vi "Append Image to Report (path).vi"(0 "report in":refnum<class "NI_HTML.lvclass">, 1 "alignment (default)":T1, 2 "MS Office parameters":T2, 7 "path or URL of image":path, 9 "caption or alternative string":string, 11 "error in (no error)":errorcluster) -> (4 "report out":refnum<class "NI_HTML.lvclass">, 8 "start out (Word)":i32, 10 "end out (Word)":i32, 15 "error out":errorcluster)   [LabVIEW 2017, in "NI_HTML.lvclass"]
doc: "For an HTML report, the VI embeds a link to an image into the report. For a standard report, the VI appends the image from a file. You can wire either a path to the image or a string that contains the image URL to this polymorphic VI. The data type you wire to the <B>path or URL of image</B> input determines the polymorphic instance to use."
uses:
  <vilib>/Utility/NIReport.llb/HTML/NI_HTML.lvclass
  <vilib>/Utility/NIReport.llb/HTML Report Image Alignment.ctl
  <vilib>/Utility/NIReport.llb/HTML/NI_HTML.lvclass/NI_HTML.ctl
  <vilib>/Utility/NIReport.llb/NI_ReportGenerationCore.lvlib
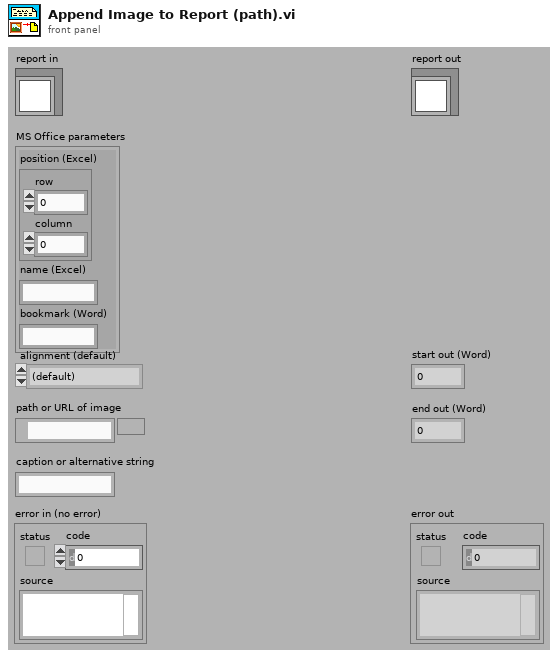
[diagram p1: front panel]
types:
  T1 = typedef "NI_ReportGenerationCore.lvlib/HTML Report Image Alignment.ctl" = enum16{"(default)", "LEFT", "RIGHT", "TOP", "TEXTTOP", "MIDDLE", "ABSMIDDLE", "BASELINE", "BOTTOM", "ABSBOTTOM"}
  T2 = cluster{"position (Excel)":cluster{"row":i32, "column":i32}, "name (Excel)":string, "bookmark (Word)":string}
  T3 = typedef "NI_ReportGenerationCore.lvlib/HTML Report Data.ctl" = cluster{"Body Text":string, "Font Tag":string, "Title Text":string, "Header Text":string, "Footer Text":string, "Image List":path[]}
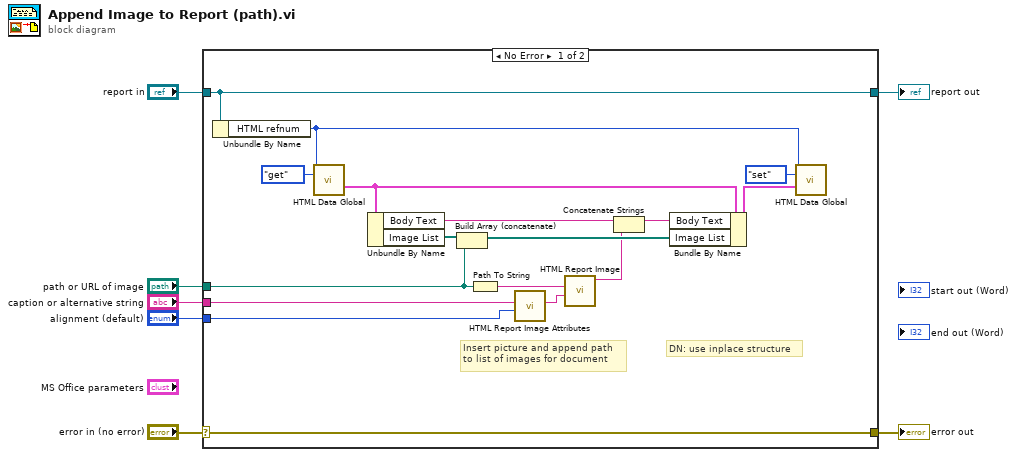
[diagram p0: block diagram]
diagram:
  n1 = case shown="No Error" "error in (no error)" {
    selector: "error in (no error)" -> [w24 w26]
    tunnel: [w24 w26] -> w6
    tunnel: [w15 w25] -> w4
    tunnel: "report in" -> [w15 w25]
    tunnel: "caption or alternative string" -> [w20 _]
    tunnel: "path or URL of image" -> [w19 _]
    tunnel: "alignment (default)" -> [w18 _]
    frame No Error {
      # "DN: use inplace structure"
      # "Insert picture and append path\nto list of images for document"
      n2 = Unbundle By Name(w15) -> ("HTML refnum"=w8:u32)
      n3 = call <vilib>:"HTML Data Global.vi"("HTML refnum"=w8, "menu"=enum16{"init", "get", "set", "delete"}."get") -> ("HTML report data out"=w13:T3)  [unwired: 1 in, 12 out]
      n4 = Unbundle By Name(w13) -> ("Body Text"=w14:string, "Image List"=w17:path[])
      n5 = Build Array (concatenate)(w17, w19) -> (w12:path[])
      n6 = Path To String(path=w19) -> (string=w21:string)
      n7 = call <vilib>:"HTML Report Image Attributes.vi"("alignment (default)"=w18, "alt - alternative string"=w20) -> ("attributes out"=w22:string)  [unwired: 5 out]
      n8 = call <vilib>:"HTML Report Image.vi"("image attributes"=w22, "src - URL of image to embed"=w21) -> ("HTML out"=w11:string)  [unwired: 2 in, 7 out]
      n9 = Concatenate Strings(w14, w11) -> (w23:string)
      n10 = Bundle By Name(cluster=w13, "Body Text"=w23, "Image List"=w12) -> (w9:T3)
      n11 = call <vilib>:"HTML Data Global.vi"("HTML refnum"=w8, "menu"=enum16{"init", "get", "set", "delete"}."set", "HTML report data in"=w9) -> ()  [unwired: 13 out]
    }
    frame Error {
    }
  }
  "error out" <- w6
  "report out" <- w4
